vi "parse listbox name.vi"(11 "formatted name":string) -> (2 "display":string, 3 "ID":string)   [LabVIEW 2013, in "Standard Engine Editor Node.lvclass"]
uses:
  Standard Engine Editor Node.lvclass
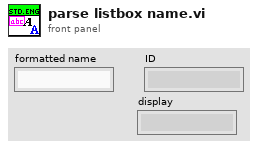
[diagram p1: front panel]
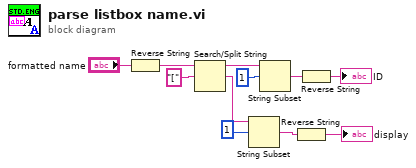
[diagram p0: block diagram]
diagram:
  n1 = Reverse String(1:"formatted name") -> (0:w6:string)
  n2 = Search/Split String(string=w6, search string/char (-)="[") -> (substring before match=w8:string, match + rest of string=w4:string)  [unwired: 1 in, 1 out]
  n3 = String Subset(string=w4, offset (0)=1) -> (substring=w2:string)  [unwired: 1 in]
  n4 = String Subset(string=w8, offset (0)=1) -> (substring=w10:string)  [unwired: 1 in]
  n5 = Reverse String(1:w2) -> (0:→"display":string)
  n6 = Reverse String(1:w10) -> (0:→"ID":string)
